vi "Direct Message Sent.vi"(8 "error in (no error)":errorcluster, 10 "Message":T1, 11 "Server in":refnum<class "Server.lvclass">) -> (0 "error out":errorcluster, 3 "Server out":refnum<class "Server.lvclass">)   [LabVIEW 2020, in "Server.lvlib" / "Server.lvclass"]
uses:
  Server.lvclass
  Controls/Message Control.ctl
  Server.lvclass/Server.ctl
  Chat Window Model/Chat Window Model Messages/New Message Msg/New Message Msg.lvclass/New Message Msg.ctl
  <vilib>/ActorFramework/Message Enqueuer/Message Enqueuer.lvclass/Message Enqueuer.ctl
  <vilib>/ActorFramework/Message Enqueuer/Enqueue.vi
  Chat Window Model/Chat Window Model Messages/New Message Msg/New Message Msg.lvclass
  C:/Program Files/National Instruments/LabVIEW 2020/vi.lib/ActorFramework/Message/Message.lvclass
  <vilib>/ActorFramework/Message Priority Queue/Priority Enqueue.vi
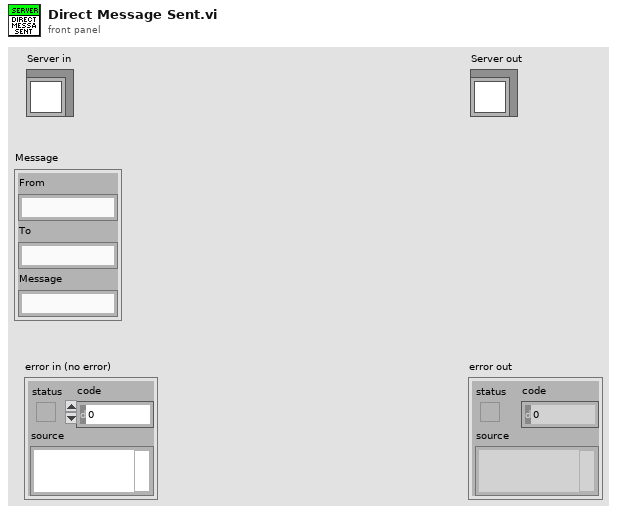
[diagram p1: front panel]
types:
  T1 = typedef "Message Control.ctl" = cluster{"From":string, "To":string, "Message":string}
  T2 = map{string, cluster{"Enqueuer":refnum<class "Message Enqueuer.lvclass">, "Status":string}}
  T3 = cluster{"Enqueuer":refnum<class "Message Enqueuer.lvclass">, "Status":string}
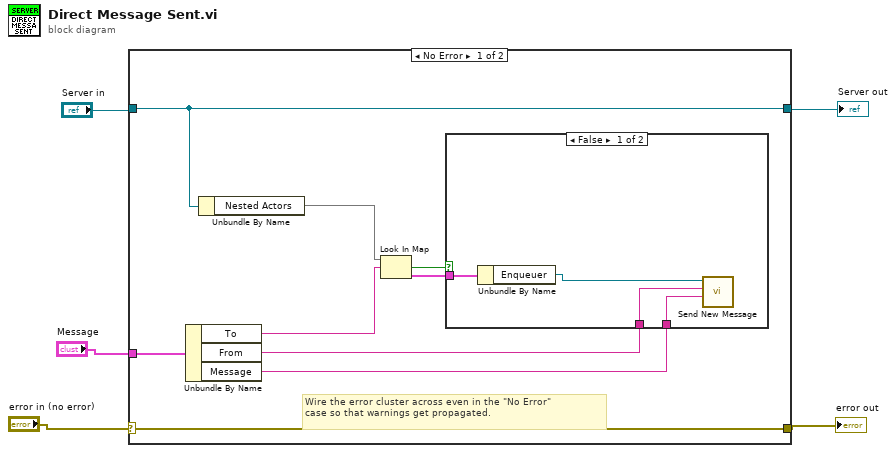
[diagram p0: block diagram]
diagram:
  n1 = case shown="No Error" "error in (no error)" {
    selector: "error in (no error)" -> [w14 w20]
    tunnel: [w14 w20] -> w1
    tunnel: [w13 w19] -> w4
    tunnel: "Server in" -> [w13 w19]
    tunnel: "Message" -> [w12 _]
    frame No Error {
      # "Wire the error cluster across even in the \"No Error\"\ncase so that warnings get propagated."
      n2 = Unbundle By Name(w12) -> ("To"=w8:string, "From"=w11:string, "Message"=w10:string)
      n3 = Unbundle By Name(w13) -> ("Nested Actors"=w9:T2)
      n4 = Look In Map(map=w9, key=w8) -> (key not found?=w7:bool, value=w6:T3)  [unwired: 1 in]
      n5 = case shown="False" w7 {
        tunnel: w11 -> [w18 _]
        tunnel: w10 -> [w17 _]
        tunnel: w6 -> [w16 _]
        frame False {
          n6 = Unbundle By Name(w16) -> ("Enqueuer"=w15:refnum<class "Message Enqueuer.lvclass">)
          n7 = call "Send New Message.vi"("New Message"=w17, "From"=w18, "Message Enqueuer"=w15) -> ()  [unwired: 7 in, 2 out]
        }
        frame True {
        }
      }
    }
    frame Error {
    }
  }
  "error out" <- w1
  "Server out" <- w4
